vi "huan-.vi"(9 "缓起清零输入":bool, 10 "循环数(100)输入":dbl=100.0, 11 "值输入":dbl) -> (3 "数值":dbl)   [LabVIEW 2017]
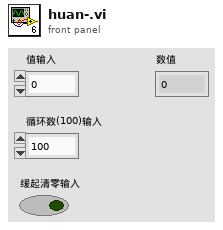
[diagram p1: front panel]
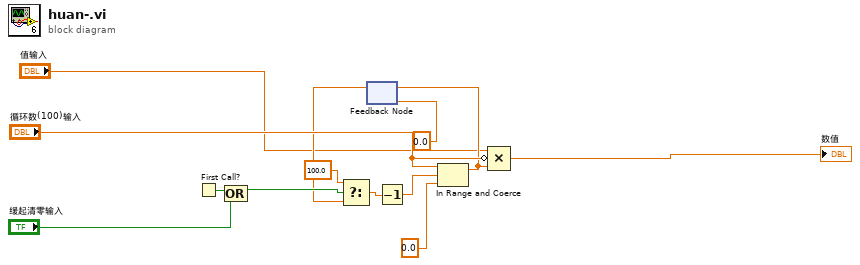
[diagram p0: block diagram]
diagram:
  n1 = First Call?() -> (First Call?: T/F=w7:bool)
  n2 = Compound Arithmetic op=OR ("复合运算")(w7, "缓起清零输入") -> (w12:bool)
  n3 = feedback #1(0.0) -> (w6:dbl)
  n4 = Select(t=100.0, s=w12, f=w6) -> (s? t:f=w9:dbl)
  n5 = Decrement(x=w9) -> (x-1=w4:dbl)
  n6 = In Range and Coerce(upper limit="循环数(100)输入", x=w4, lower limit=0.0 ("下限")) -> (coerced(x)=w10:dbl)  [unwired: 1 out]
  n7 = feedback-in #1(w10) -> ()
  n8 = Compound Arithmetic op=MULTIPLY("值输入", invert "循环数(100)输入", w10) -> (→"数值":dbl)
